vi "Dashboard Main.vi"() -> ()   [LabVIEW 2019]
uses:
  <vilib>/Utility/miscctls.llb/LVRowAndColumnTypeDef.ctl
  <vilib>/event_ctls.llb/eventvkey.ctl
  <vilib>/Rock Robotics/Network Tables/NT Read Numeric Array.vi
  <vilib>/Rock Robotics/WPI/Dashboard/WPI_DashboardLogging Global.vi
  <vilib>/Rock Robotics/Network Tables/NT Read Boolean.vi
panel:
  in  "Camera Settings Right":T1={"Frame Rate"=30, "Compression"=30, "Size"=1, "DB Camera Config"=FALSE} {"Frame Rate" scale=1.0..30.0; "Compression" scale=100.0..-1.0; "Size" items=["640x480", "320x240", "160x120"]}
  in  "Camera Name Right":string(combo)="No Camera Selection"
  out "Camera Perf":string
  in  "Camera Settings":T1={"Frame Rate"=30, "Compression"=30, "Size"=1, "DB Camera Config"=FALSE} {"Frame Rate" scale=1.0..30.0; "Compression" scale=100.0..-1.0; "Size" items=["640x480", "320x240", "160x120"]}
  in  "TCP":refnum<k5>
  in  "Rec Mode":enum32{"Stop", "Record", "Playback"}(radio)
  out "Robot IP":string
  out "Image Message":string="Timeout in Camera Communications"
  in  "Dashboard Tab":T2(tab)
  out "Vision Enabled":bool
  in  "Select Auto":string(combo)="Select Autonomous ..."
  out "NT Connection":bool
  out "MotorChart R":cluster{"Numeric":dbl, "Numeric":dbl}(graph)
  out "MotorChart L":cluster{"Numeric":dbl, "Numeric":dbl}(graph)
  out "MotorSliders R":cluster{"MotorSlide1":dbl, "MotorSlide2":dbl} {"MotorSlide2" scale=-1.0..1.0 scale format="%#_2e"; "MotorSlide1" scale=-1.0..1.0 scale format="%#_2e"}
  out "MotorSliders L":cluster{"MotorSlide1":dbl, "MotorSlide2":dbl} {"MotorSlide2" scale=-1.0..1.0 scale format="%#_2e"; "MotorSlide1" scale=-1.0..1.0 scale format="%#_2e"}
  out "JS1 Z":dbl(slide) scale=-1.0..1.0 scale format="%#_2e"
  out "JS1 Graph":cluster{"X":dbl, "Y":dbl}[](graph)
  out "JS1 Buttons":T3
  out "JS2 Z":dbl(slide) scale=-1.0..1.0 scale format="%#_2e"
  out "JS2 Graph":cluster{"X":dbl, "Y":dbl}[](graph)
  out "JS2 Buttons":T3
  out "Mode":T4(ring)=enum."Auto Disabled"
  out "Right Camera Perf":cluster{"Bandwidth (Mbps)":dbl, "FPS":dbl}
  out "Top RPM":dbl caption="DB/String 1"
  out "Bottom RPM":dbl caption="DB/String 1"
  out "Target Distance":dbl
  out "Camera Image Right":T5(plugin-control)
  out "Skew":dbl caption="DB/String 1"
  out "Area":dbl caption="DB/String 1"
  out "Offset X":dbl
  out "Offset Y":dbl
  in  "Test Slider":dbl(slide) scale=0.0..100.0 scale format="%#_3g"
  in  "On/Off":bool caption="Solenoid"
  in  "Test Name":u16(ring) items=["Select the test to run..."]
  in  "Test Tree":string(tree)
  in  "Motor":cluster{"Value":dbl, "Enable":bool} {"Value" scale=-1.0..1.0 scale format="%#_3g"}
  out "Progress":T6 {"Test Progress" scale=0.0..100.0}
  in  "Rev/Fwd":cluster{"Forward":bool, "Reverse":bool}
  in  "Test Ring":u16(ring) items=["Monochrome", "Color"]
  out "Cmd Status":string
  in  "Execute Command":bool
  in  "Command Params":string[][](table)
  in  "Command Selection":i32(listbox)
  in  "CheckList":i32(listbox)
  out "Tree":string(tree)
  out "Camera Image":T5(plugin-control)
  out "Background":bool
  in  "Camera Name":string(combo)="No Camera Selection"
  # "HW"
  # "HW"
  # "Drive Motors"
  # "Front"
  # "Operator 1"
  # "Operator 2"
  # "Right"
  # "Left"
  # "Back"
  # "This tab is a great place for autonomous settings and robot-specific values.\nPlace controls and indicators inside this tab and match name to\nDashboard Variables on robot. You can also delete this comment."
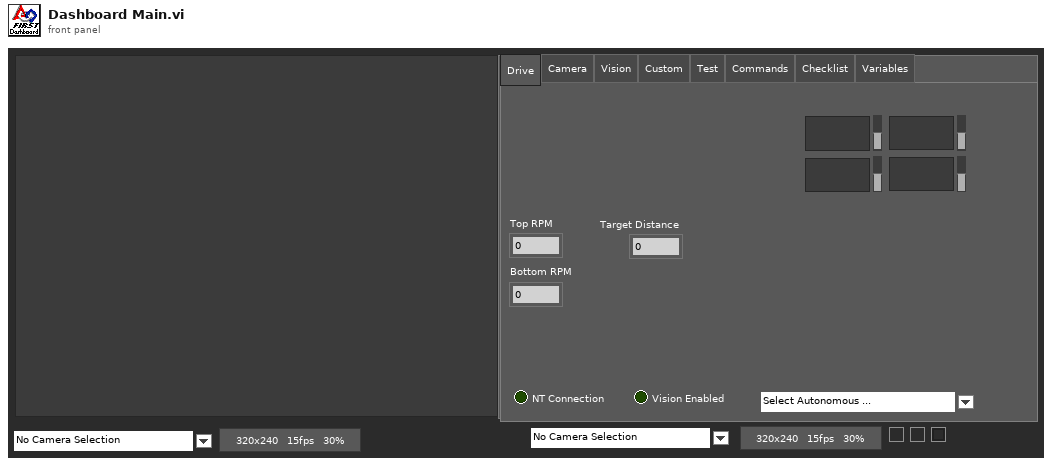
[diagram p1: front panel]
types:
  T1 = cluster{"Frame Rate":i32, "Compression":i32, "Size":u16, "DB Camera Config":bool}
  T2 = enum32{"Drive", "Camera", "Vision", "Custom", "Test", "Commands", "Checklist", "Variables"}
  T3 = cluster{bool, bool, bool, bool, bool, bool, bool, bool, bool, bool, bool, bool}
  T4 = enum8{"Tele-Op Disabled", "Tele-Op Enabled", "Auto Disabled", "Auto Enabled", "Test Disabled", "Test Enabled", "Disconnected", "No Code", "E-Stop"}
  T5 = typedef "IMAQ Image.ctl" = refnum<image>
  T6 = cluster{"Test Progress":u8, "Test Progress Text":string}
  T7 = cluster{"Save Path":path, "Interval (s)":dbl, "Keep":i32}
  T8 = enum32{"Drive", "Camera", "Basic", "Custom", "Test", "Commands", "Checklist", "Variables"}
  T9 = typedef "Image Type" = u32
  T10 = cluster{"IDs":cluster{"RPC field ID":u16, "Unique ID":u16}, "String":string}
  T11 = cluster{"Camera Image":refnum<vi>, "Dashboard Tab":refnum<vi>, "Background":refnum<vi>, "Rec Mode":refnum<vi>, "Test Slider":refnum<vi>, "On/Off ":refnum<vi>, "Test Ring":refnum<vi>, "Rev/Fwd":refnum<vi>, "Test Name":refnum<vi>, "Motor":refnum<vi>, "Progress":refnum<vi>, "CheckList":refnum<vi>, "Tree":refnum<vi>, "Test Tree":refnum<vi>, "Command Params":refnum<vi>, "Command Selection":refnum<vi>, "Execute Command":refnum<vi>, "Cmd Status":refnum<vi>, "Camera Settings":refnum<vi>, "Camera Name":refnum<vi>, "Camera Perf":refnum<vi>, "Camera Settings Right":refnum<vi>, "Camera Name Right":refnum<vi>, "Camera Image Right":refnum<vi>}
  T12 = cluster{"Global Rectangle":i32[], "Contours":cluster{"Contour Type":u32, "ROI Type":u32, "Points":i32[]}[]}
  T13 = cluster{"Camera Name Right":string, string, "Saved DB Images Info":cluster{"Save Path":path, "Interval (s)":dbl, "Keep":i32}}
  T14 = cluster{"Error Strings":string, "Disable Counts":cluster{u16, u16}, "Rail Faults":cluster{u16, u16, u16}, "Robot IP":string, "DB Mode":u8, "Event Info":cluster{"Name":string, "Type":u8, "Number":u16, "Replay":u8}}
  T15 = cluster{"Storage":cluster{"Disk Free":u64, "RAM Block":u32, "RAM free":u32}, "CPU Utilization":cluster{"CPU % ISR":sgl, "CPU % Time Crit":sgl, "CPU % Timed Str":sgl, "CPU % High":sgl, "CPU % Above":sgl, "CPU % Normal":sgl, "CPU % Low":sgl}, "CAN":cluster{"% Bus Utilization":sgl, "Bus Off Cnt":u32, "TX_FIFO Full Cnt":u32, "Receive Error Cnt":u8, "Transmit Error Cnt":u8}, "HID":cluster{"HID Outputs":u32, "Rumble Low":u16, "Rumble High":u16}[]}
  T16 = cluster{"Status bits":cluster{"Test Mode":bool, "Autonomous":bool, "Enabled":bool, "Code Start":bool, "Brownout":bool, "Reserved 2":bool, "Reserved 3":bool, "E-Stop":bool}, "Code Trace":cluster{"Disabled":bool, "TeleOp":bool, "Auto":bool, "Test":bool}, "Controller Type":enum16{"unknown", "cRIO", "roboRio"}, "Code?":enum16{"unknown", "noCode", "code"}, "Battery V":dbl}
  T17 = cluster{"Control Bits":cluster{"TestMode":bool, "Autonomous":bool, "Enabled":bool, "FMS Present":bool, bool, bool, bool, "E-Stop":bool}, "Team Station ":u8, "Countdown":sgl, "Joystick Values":cluster{"Axes":dbl[], "Buttons":bool[], "POVs":i16[]}[]}
  T18 = cluster{"Axes":dbl[], "Buttons":bool[], "POVs":i16[]}[]
  T19 = cluster{"Axes":dbl[], "Buttons":bool[], "POVs":i16[]}
  T20 = cluster{"Buttons[0]":bool, "Buttons[1]":bool, "Buttons[2]":bool, "Buttons[3]":bool, "Buttons[4]":bool, "Buttons[5]":bool, "Buttons[6]":bool, "Buttons[7]":bool, "Buttons[8]":bool, "Buttons[9]":bool, "Buttons[10]":bool, "Buttons[11]":bool}
  T21 = cluster{"Camera Name":string, string, "Saved DB Images Info":cluster{"Save Path":path, "Interval (s)":dbl, "Keep":i32}}
  T22 = cluster{"Operation":enum16{"Update", "Clear"}, "Color Box":u32}[]
  T23 = typedef "eventvkey.ctl" = enum16{"ASCII", "Enter", "Return", "Shift", "Ctrl", "Alt", "Cmd", "Opt", "Caps", "NumLock", "Clear", "Break", "Up", "Down", "Left", "Right", "Insert", "Delete", "Home", "End", "PageUp", "PageDown", "Escape", "Help", "Pause", "ScrollLock", "F1", "F2", "F3", "F4", "F5", "F6", "F7", "F8", "F9", "F10", "F11", "F12", "F13", "F14", "F15", "F16", "F17", "F18", "F19", "F20", "F21", "F22", "F23", "F24", "Play", "VolumeUp", "VolumeDown", "Mute", "Two Byte Char"}
  T24 = cluster{"Image Size":bool, "Image Type":bool, "Pixel Value":bool, "ROI Information":bool, "Zoom Factor":bool}
  T25 = cluster{"Operation":enum16{"Update", "Clear"}, "Color Box":u32}
  T26 = typedef "LVRowAndColumnTypeDef.ctl" = cluster{"Row":i32, "Column":i32}
  T27 = cluster{"Shift":bool, "Ctrl":bool, "Alt":bool, "Cmd":bool, "Opt":bool}
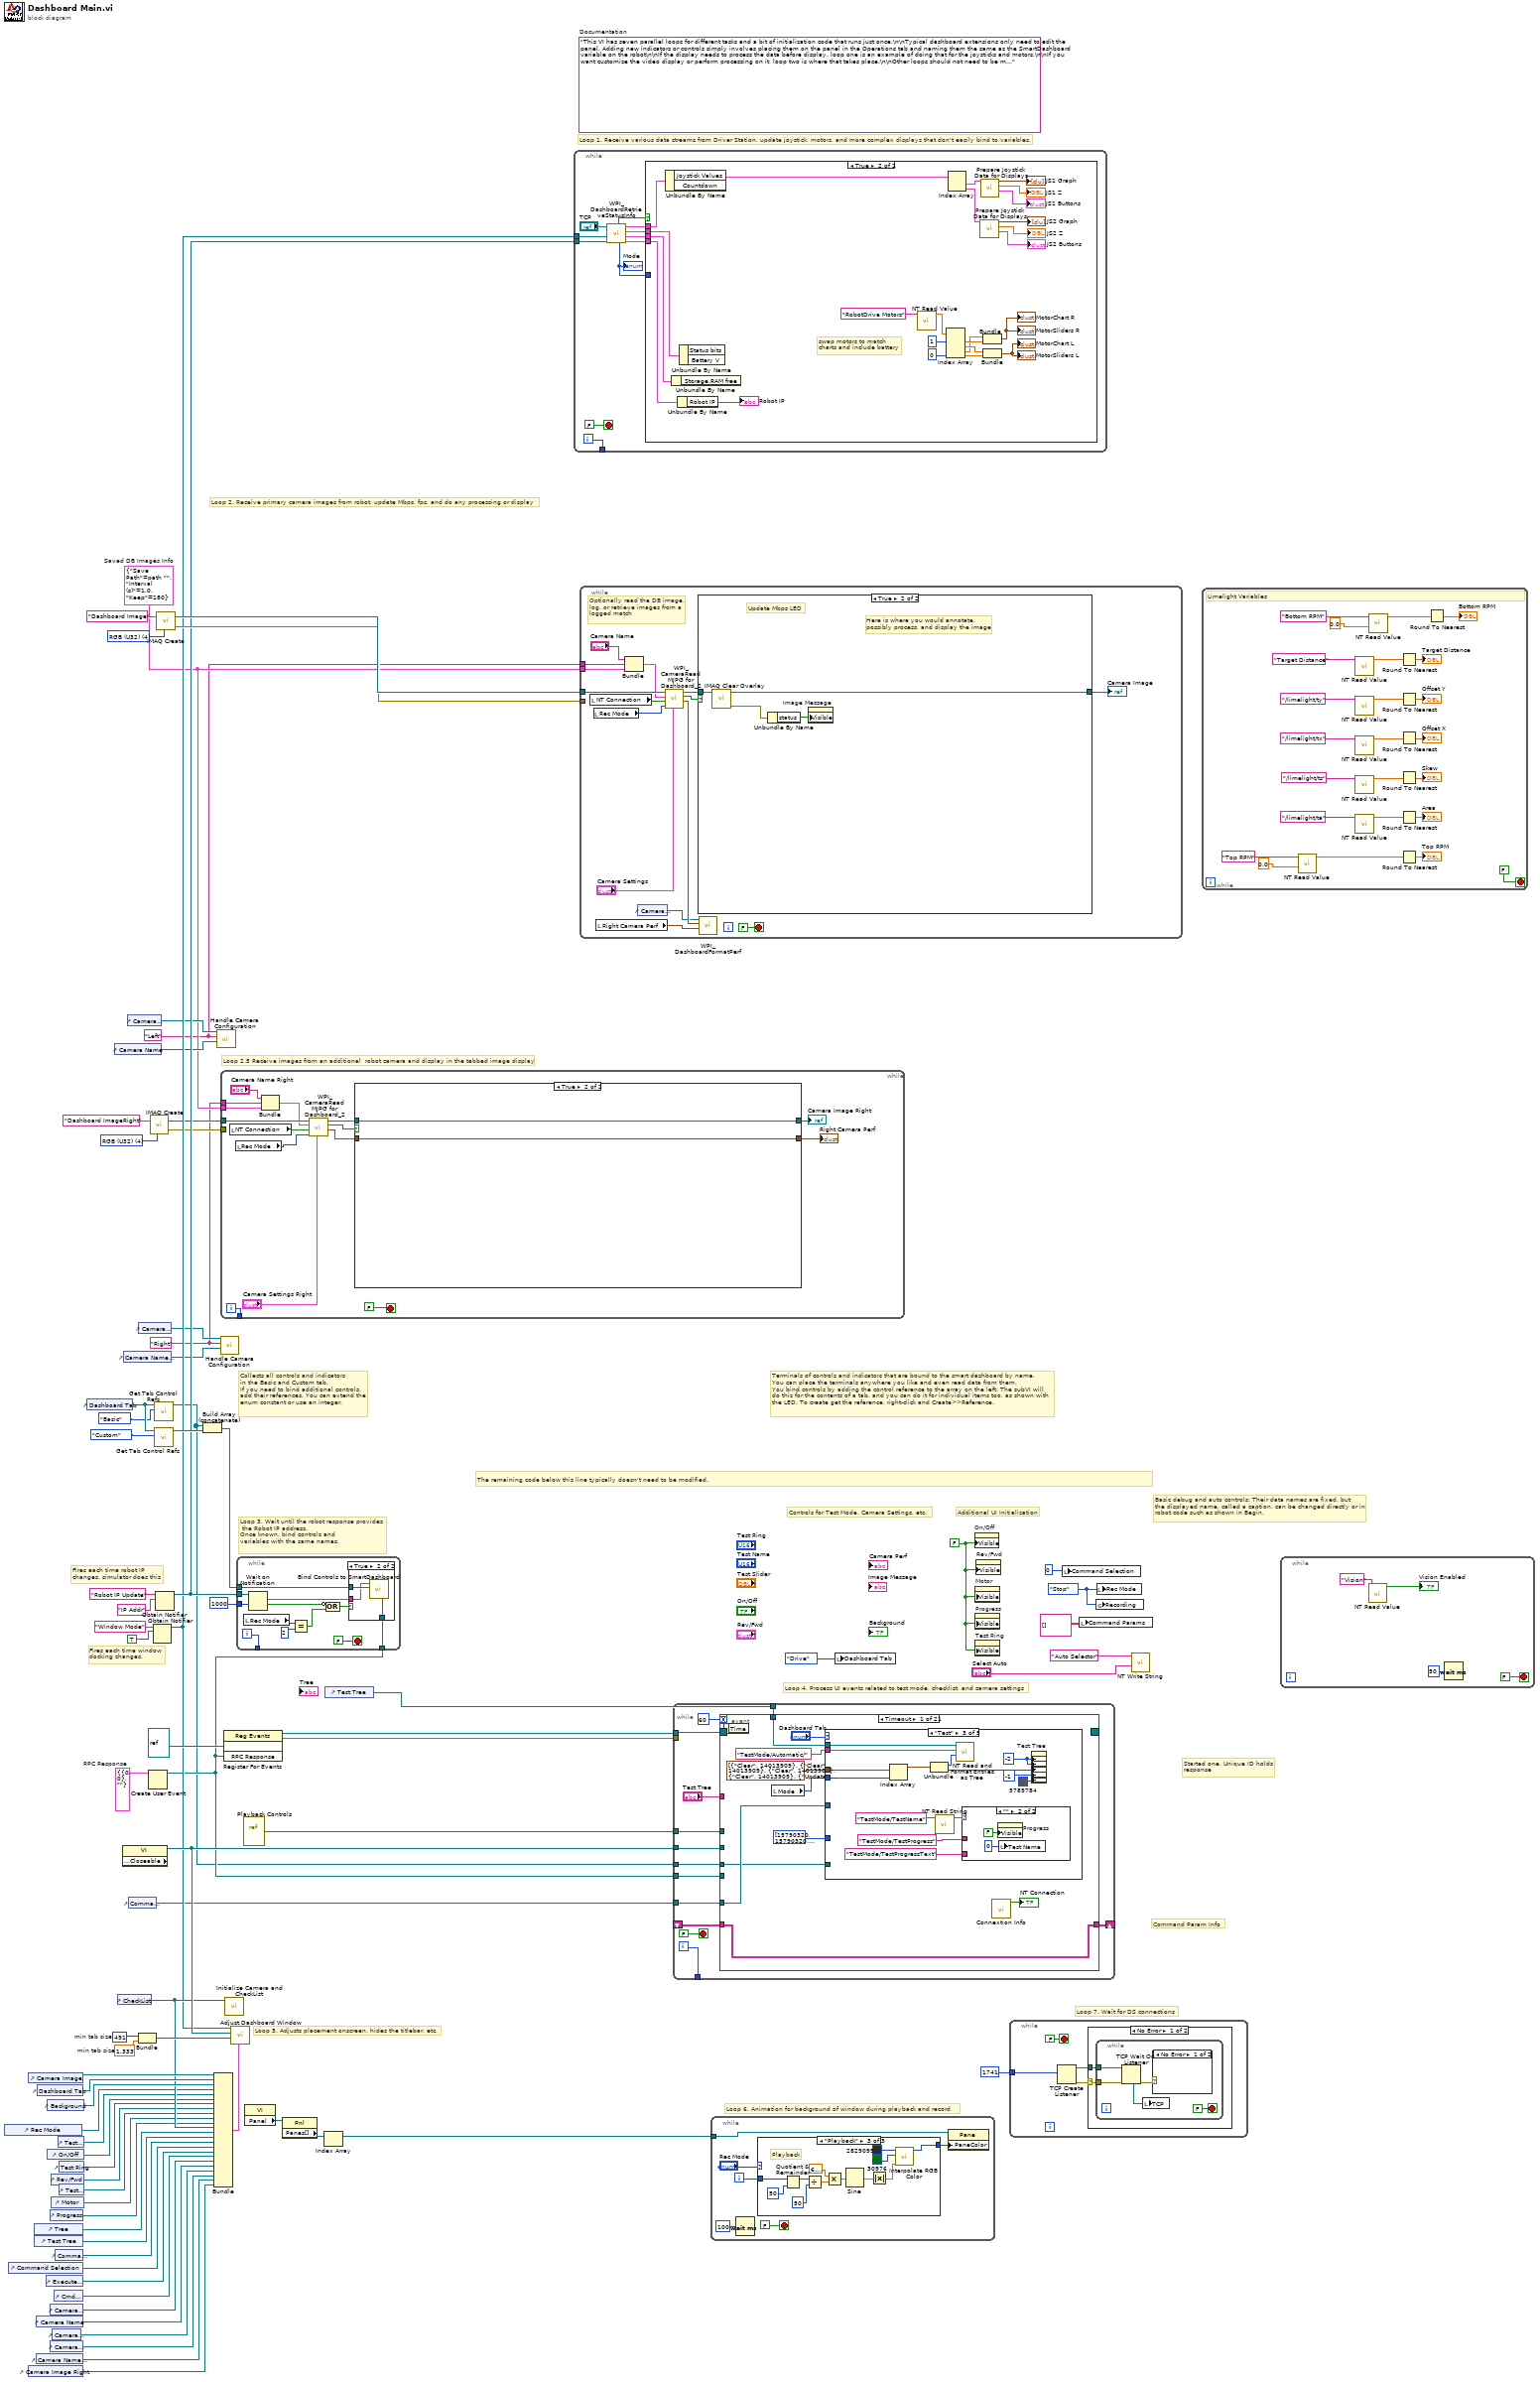
[diagram p0: block diagram]
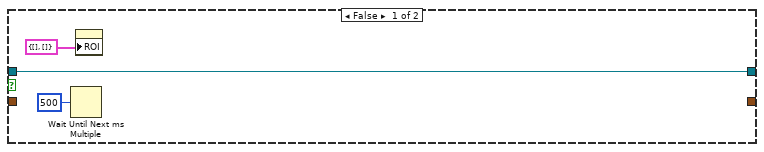
[diagram p2: hidden frame]
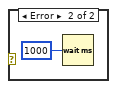
[diagram p3: hidden frame]
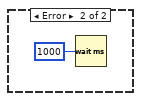
[diagram p4: hidden frame]
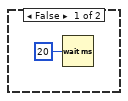
[diagram p5: hidden frame]
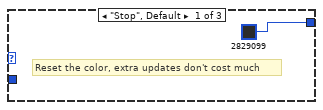
[diagram p6: hidden frame]
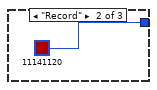
[diagram p7: hidden frame]
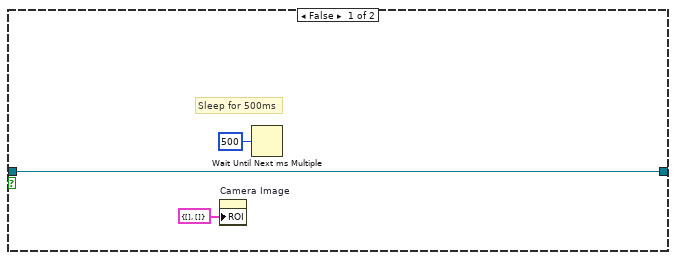
[diagram p9: hidden frame]
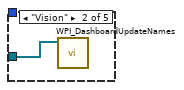
[diagram p11: hidden frame]
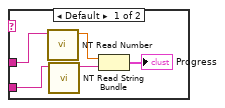
[diagram p12: hidden frame]
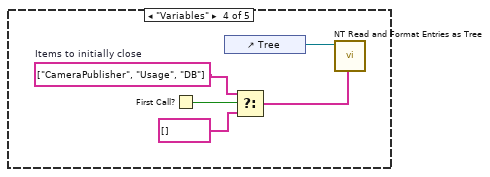
[diagram p13: hidden frame]
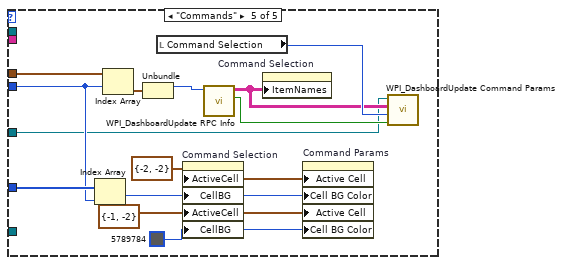
[diagram p14: hidden frame]
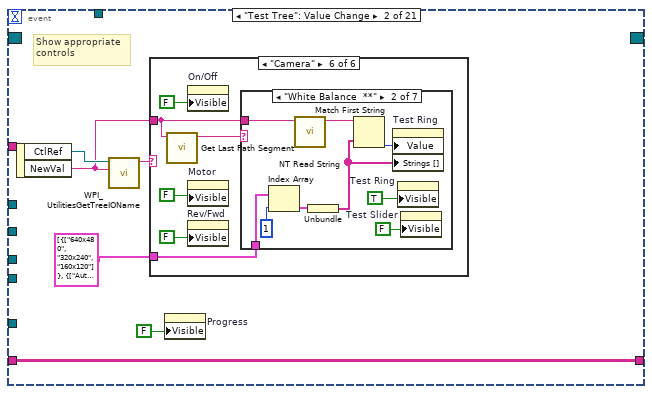
[diagram p15: hidden frame]
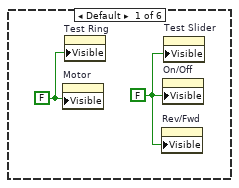
[diagram p16: hidden frame]
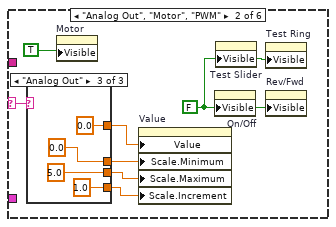
[diagram p17: hidden frame]
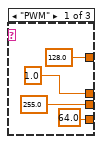
[diagram p18: hidden frame]
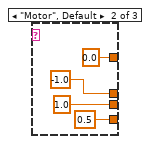
[diagram p19: hidden frame]
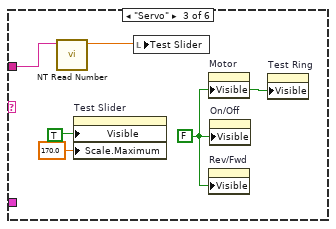
[diagram p20: hidden frame]
diagram:
  w4 = T7 {"Save Path"=path "", "Interval (s)"=1.0, "Keep"=180}  # Saved DB Images Info
  w3 = "Right"
  w2 = "Left"
  w14 = T9 4 items=["Grayscale (U8)", "Grayscale (I16)", "Grayscale (SGL)", "Complex (CSG)", "RGB (U32)", "HSL (U32)", "RGB (U64)"] ("Image Type")
  w30 = T10 {"IDs"={"RPC field ID"=0, "Unique ID"=0}, "String"=""}  # RPC Response
  w52 = 491  # min tab size
  w51 = 1.333  # min tab size
  w59 = enum32{"Stop", "Record", "Playback"}."Stop" ("Rec Mode")
  w36 = FALSE ("Visible")
  (unwired) "This VI has seven parallel loops for different tasks and a bit of initialization code that runs just once.\n\nTypical dashboard extensions only need to edit the panel. Adding new indicators or controls simply involves placing them on the panel in the Operations tab and naming them the same as the SmartDashboard variable on the robot\n\nIf the display needs to process the data before display, loop one is an example of doing that for the joysticks and motors.\n\nIf you want customize the video display or perform processing on it, loop two is where that takes place.\n\nOther loops should not need to be modified. They are pretty standard, and document the task they perform."  # Documentation
  w76 = T9 4 items=["Grayscale (U8)", "Grayscale (I16)", "Grayscale (SGL)", "Complex (CSG)", "RGB (U32)", "HSL (U32)", "RGB (U64)"] ("Image Type")
  # "Loop 2.5 Receive images from an additional  robot camera and display in the tabbed image display"
  # "Command Param Info"
  # "Started one, Unique ID holds\nresponse"
  # "Loop 7. Wait for DS connections"
  # "Basic debug and auto controls: Their data names are fixed, but\nthe displayed name, called a caption, can be changed directly or in\nrobot code such as shown in Begin."
  # "Controls for Test Mode, Camera Settings, etc."
  # "Additional UI Initialization"
  # "Loop 6. Animation for background of window during playback and record"
  # "Fires each time robot IP\nchanges, simulator does this"
  # "Fires each time window\ndocking changes."
  # "Collects all controls and indicators\nin the Basic and Custom tab.\nIf you need to bind additional controls,\nadd their references. You can extend the\nenum constant or use an integer."
  # "The remaining code below this line typically doesn't need to be modified."
  # "Loop 4. Process UI events related to test mode, checklist, and camera settings"
  # "Terminals of controls and indicators that are bound to the smart dashboard by name.\nYou can place the terminals anywhere you like and even read data from them.\nYou bind controls by adding the control reference to the array on the left. The subVI will\ndo this for the contents of a tab, and you can do it for individual items too, as shown with\nthe LED. To create get the reference, right-click and Create>>Reference."
  # "Loop 3. Wait until the robot response provides\n the Robot IP address.\nOnce known, bind controls and\nvariables with the same names."
  # "Loop 5. Adjusts placement onscreen, hides the titlebar, etc."
  # "Loop 1. Receive various data streams from Driver Station, update joystick, motors, and more complex displays that don't easily bind to variables."
  # "Loop 2. Receive primary camera images from robot, update Mbps, fps, and do any processing or display"
  n1 = control-ref of="Rec Mode"() -> (w42:refnum<vi>)
  n2 = control-ref of="Command Selection"() -> (w29:refnum<vi>)
  n3 = control-ref of="Camera Image Right"() -> (w7:refnum<vi>)
  n4 = control-ref of="Camera Image"() -> (w54:refnum<vi>)
  n5 = control-ref of="Tree"() -> (w46:refnum<vi>)
  n6 = control-ref of="Test Tree"() -> (w45:refnum<vi>)
  n7 = control-ref of="Camera Name"() -> (w20:refnum<vi>)
  n8 = control-ref of="Camera Name Right"() -> (w8:refnum<vi>)
  n9 = control-ref of="Dashboard Tab"() -> (w53:refnum<vi>)
  n10 = control-ref of="Execute Command"() -> (w31:refnum<vi>)
  n11 = control-ref of="Background"() -> (w49:refnum<vi>)
  n12 = control-ref of="On/Off"() -> (w40:refnum<vi>)
  n13 = control-ref of="Progress"() -> (w37:refnum<vi>)
  n14 = control-ref of="Camera Settings"() -> (w21:refnum<vi>)
  n15 = control-ref of="Camera Settings Right"() -> (w9:refnum<vi>)
  n16 = control-ref of="Rev/Fwd"() -> (w38:refnum<vi>)
  n17 = control-ref of="Motor"() -> (w43:refnum<vi>)
  n18 = control-ref of="Camera Perf"() -> (w19:refnum<vi>)
  n19 = control-ref of="Cmd Status"() -> (w25:refnum<vi>)
  n20 = control-ref of="Command Params"() -> (w32:refnum<vi>)
  n21 = control-ref of="Test Slider"() -> (w41:refnum<vi>)
  n22 = control-ref of="Test Ring"() -> (w39:refnum<vi>)
  n23 = control-ref of="Test Name"() -> (w44:refnum<vi>)
  n24 = control-ref of="Dashboard Tab"() -> (w57:refnum<vi>)
  n25 = control-ref of="Camera Name"() -> (w22:refnum<vi>)
  n26 = control-ref of="CheckList"() -> (w47:refnum<vi>)
  n27 = property class="VI" props=["Front Panel.Closeable"]() -> (reference out=w58:refnum<vi>)  [unwired: 2 in, 2 out]
  n28 = control-ref of="Camera Name Right"() -> (w10:refnum<vi>)
  n29 = control-ref of="Camera Settings"() -> (w23:refnum<vi>)
  n30 = control-ref of="Command Params"() -> (w24:refnum<vi>)
  n31 = control-ref of="Camera Settings Right"() -> (w11:refnum<vi>)
  n32 = Bundle("min tab size"=w52, "min tab size"=w51) -> (w50:cluster{"min tab size":i32, "min tab size":dbl})  [unwired: 1 in]
  n33 = Create User Event(user event datatype=w30) -> (user event=w26:refnum<user-event>)  [unwired: 1 in, 1 out]
  n34 = call "IMAQ Create"("Image Name"="Dashboard ImageRight", "Image Type"=w14) -> ("New Image"=w13:T5, "error out"=w12:errorcluster)  [unwired: 2 in, 1 out]
  n35 = Obtain Notifier(name (unnamed)="Window Mode", notification data type=TRUE) -> (notifier out=w34:refnum<notifier>)  [unwired: 2 in, 2 out]
  n36 = call <vilib>:"Get Tab Control Refs.vi"("Page Index"=T8."Basic" ("Dashboard Tab"), "TabControl in"=w57) -> ("ControlsOnPage"=w18:refnum<vi>[])  [unwired: 9 in]
  n37 = call <vilib>:"Get Tab Control Refs.vi"("Page Index"=T8."Custom" ("Dashboard Tab"), "TabControl in"=w57) -> ("ControlsOnPage"=w56:refnum<vi>[])  [unwired: 9 in]
  n38 = Obtain Notifier(name (unnamed)="Robot IP Update", notification data type="IP Addr" ("name (unnamed)")) -> (notifier out=w35:refnum<notifier>)  [unwired: 2 in, 2 out]
  n39 = call "IMAQ Create"("Image Name"="Dashboard Image", "Image Type"=w76) -> ("New Image"=w74:T5, "error out"=w73:errorcluster)  [unwired: 2 in, 1 out]
  n40 = Build Array (concatenate)(w18, w56) -> (w55:refnum<vi>[])
  n41 = Bundle("Camera Image"=w54, "Dashboard Tab"=w53, "Background"=w49, "Rec Mode"=w42, "Test Slider"=w41, "On/Off"=w40, "Test Ring"=w39, "Rev/Fwd"=w38, "Test Name"=w44, "Motor"=w43, "Progress"=w37, "CheckList"=w47, "Tree"=w46, "Test Tree"=w45, "Command Params"=w32, "Command Selection"=w29, "Execute Command"=w31, "Cmd Status"=w25, "Camera Settings"=w21, "Camera Name"=w20, "Camera Perf"=w19, "Camera Settings Right"=w9, "Camera Name Right"=w8, "Camera Image Right"=w7) -> (w48:T11)  [unwired: 1 in]
  n42 = call "Handle Camera Configuration.vi"("CameraNameRef"=w22, "Display Name"=w2, "ClusterRef"=w23) -> ()  [unwired: 9 in]
  n43 = call "Handle Camera Configuration.vi"("CameraNameRef"=w10, "Display Name"=w3, "ClusterRef"=w11) -> ()  [unwired: 9 in]
  n44 = while {
    tunnel: w13 -> [w91]
    tunnel: w12 -> [_]
    tunnel: [w86] -> _
    tunnel: w4 -> [w83]
    tunnel: w3 -> [w80]
    i -> [w86]
    stop <- FALSE stop-if-true
    n45 = local read "NT Connection"() -> (w84:bool)
    n46 = local read "Rec Mode"() -> (w90:enum32{"Stop", "Record", "Playback"})
    n47 = Bundle("Camera Name Right"="Camera Name Right", w80, "Saved DB Images Info"=w83) -> (w82:T13)  [unwired: 1 in]
    n48 = call <vilib>:"WPI_CameraRead MJPG for Dashboard_2.vi"("Camera Settings"="Camera Settings Right", "Rec Mode"=w90, "NT Connection"=w84, "Capture Info"=w82, "Image in"=w91) -> ("perf info"=w78:cluster{"Bandwidth (Mbps)":dbl, "fps":dbl}, "Active"=w85:bool, "Image\\ out"=w88:T5)  [unwired: 4 in]
    n49 = case shown="True" w85 {
      tunnel: w88 -> [w93 w95]
      tunnel: [w93 w95] -> w77
      tunnel: [_ w96] -> w79
      tunnel: w78 -> [_ w96]
      frame False {
        n50 = Wait Until Next ms Multiple(millisecond multiple=u32 500) -> ()  [unwired: 1 out]
        n51 = property on="Camera Image Right" class="ImageControl"("ROI"=T12 {"Global Rectangle"=[], "Contours"=[]}) -> ()  [unwired: 2 in, 2 out]
      }
      frame True {
      }
    }
    "Right Camera Perf" <- w79
    "Camera Image Right" <- w77
  }
  n52 = register-events(refnum<vi> refnum, w26) -> (reference out=w63:refnum<event-registration>, error out=w62:errorcluster)  [unwired: 2 in]
  n53 = call "Initialize Camera and CheckList.vi"("ListBox in"=w47) -> ()  [unwired: 11 in]
  n54 = call "Adjust Dashboard Window.vi"("Sizing Refnums"=w48, "Size Constraints"=w50, "VI"=w58, "WIn Mode"=w34) -> ()  [unwired: 8 in]
  n55 = while {
    tunnel: w55 -> [w108]
    tunnel: w35 -> [w106]
    tunnel: [w104] -> _
    tunnel: u32 1000 ("milliseconds to wait") -> [w103]
    tunnel: w26 -> [w97]
    i -> [w104]
    stop <- FALSE stop-if-true
    n56 = local read "Rec Mode"() -> (w99:enum32{"Stop", "Record", "Playback"})
    n57 = Wait on Notification(notifier=w106, timeout in ms (-1)=w103) -> (notification=w105:string, timed out?=w101:bool)  [unwired: 2 in, 2 out]
    n58 = Equal?(x=w99, y=u16 2 ("Rec Mode")) -> (x = y?=w100:bool)
    n59 = Compound Arithmetic op=OR(invert w101, w100) -> (w102:bool)
    n60 = case shown="True" w102 {
      tunnel: w108 -> [_ w111]
      tunnel: w105 -> [_ w110]
      tunnel: w97 -> [_ w109]
      frame False {
      }
      frame True {
        n61 = call <vilib>:"Bind Controls to SmartDashboard.vi"("RPC ref"=w109, "Bound Control Refs"=w111, "Server IP Address"=w110) -> ()  [unwired: 9 in]
      }
    }
  }
  n62 = vi-ref "Playback Controls.vi"() -> (w64:refnum<vi>)
  n63 = property class="VI"() -> ("Panel"=w66:refnum<vi>)  [unwired: 2 in, 2 out]
  n64 = property class="Pnl"(reference=w66) -> ("Panes[]"=w67:refnum<vi>[])  [unwired: 1 in, 2 out]
  n65 = Index Array(array=w67) -> (element=w65:refnum<vi>)  [unwired: 1 in]
  n66 = control-ref of="Test Tree"() -> (w68:refnum<vi>)
  n67 = while {
    tunnel: [w121] -> _
    tunnel: w35 -> [w115]
    tunnel: w34 -> [w112]
    i -> [w121]
    stop <- FALSE stop-if-true
    n68 = call <vilib>:"WPI_DashboardRetrieveStatusInfo.vi"("Binding Refnum"=w115, "Window Mode Notifier"=w112, "TCP Cnx"="TCP") -> ("Power and Errors"=w116:T14, "Robot Metrics"=w119:T15, "Status Info"=w120:T16, "Control Info"=w117:T17, "Robot Mode"=w114:T4, "Process?"=w118:bool)  [unwired: 3 in]
    "Mode" <- w114
    n69 = case shown="True" w118 {
      tunnel: w120 -> [_ w147]
      tunnel: w119 -> [_ w146]
      tunnel: w117 -> [_ w145]
      tunnel: w116 -> [_ w144]
      tunnel: w114 -> [_ _]
      frame False {
        n70 = Wait (ms)(milliseconds to wait=u32 20) -> ()  [unwired: 1 out]
      }
      frame True {
        # "swap motors to match\ncharts and include battery"
        n71 = Unbundle By Name(w145) -> ("Joystick Values"=w135:T18)  [unwired: 1 out]
        n72 = Unbundle By Name(w146) -> ()  [unwired: 1 out]
        n73 = Unbundle By Name(w144) -> ("Robot IP"=→"Robot IP":string)
        n74 = Unbundle By Name(w147) -> ()  [unwired: 2 out]
        n75 = call-poly <vilib>:"NT Read Value.vi"("Name"="RobotDrive Motors") -> ("Numeric Array"=w125:dbl[])  [unwired: 9 in, 1 out]
        n76 = Index Array(array=w125, index #1=1, index #4=0) -> (element #1=w139:dbl, element #2=w140:dbl, element #3=w138:dbl, element #4=w143:dbl)  [unwired: 2 in]
        n77 = Index Array(array=w135) -> (element #1=w134:T19, element #2=w130:T19)  [unwired: 2 in]
        n78 = call "Prepare Joystick Data for Displays.vi"("Joystick Values"=w130) -> ("Buttons"=→"JS2 Buttons":T20, "Z Axis"=→"JS2 Z":dbl, "Cartesian Data"=→"JS2 Graph":cluster{"X axis":dbl, "X axis":dbl}[])  [unwired: 8 in]
        n79 = call "Prepare Joystick Data for Displays.vi"("Joystick Values"=w134) -> ("Buttons"=→"JS1 Buttons":T20, "Z Axis"=→"JS1 Z":dbl, "Cartesian Data"=→"JS1 Graph":cluster{"X axis":dbl, "X axis":dbl}[])  [unwired: 8 in]
        n80 = Bundle("Numeric"=w138, "Numeric"=w139) -> (→"MotorChart R" →"MotorSliders R":cluster{"Numeric":dbl, "Numeric":dbl})  [unwired: 1 in]
        n81 = Bundle("Numeric"=w140, "Numeric"=w143) -> (→"MotorChart L" →"MotorSliders L":cluster{"Numeric":dbl, "Numeric":dbl})  [unwired: 1 in]
      }
    }
  }
  n82 = while {
    tunnel: w74 -> [w161]
    tunnel: w73 -> [_]
    tunnel: w4 -> [w155]
    tunnel: w2 -> [w152]
    stop <- FALSE stop-if-true
    # "Optionally read the DB image,\nlog, or retrieve images from a\nlogged match"
    n83 = local read "NT Connection"() -> (w156:bool)
    n84 = local read "Rec Mode"() -> (w158:enum32{"Stop", "Record", "Playback"})
    n85 = local read "Right Camera Perf"() -> (w150:cluster{"Bandwidth (Mbps)":dbl, "FPS":dbl})
    n86 = Bundle("Camera Name"="Camera Name", w152, "Saved DB Images Info"=w155) -> (w154:T21)  [unwired: 1 in]
    n87 = control-ref of="Camera Perf"() -> (w149:refnum<vi>)
    n88 = call <vilib>:"WPI_CameraRead MJPG for Dashboard_2.vi"("Camera Settings"="Camera Settings", "Rec Mode"=w158, "NT Connection"=w156, "Capture Info"=w154, "Image in"=w161) -> ("perf info"=w151:cluster{"Bandwidth (Mbps)":dbl, "fps":dbl}, "Active"=w159:bool, "Image\\ out"=w160:T5)  [unwired: 4 in]
    n89 = case shown="True" w159 {
      tunnel: w160 -> [w164 w167]
      tunnel: [w164 w166] -> w148
      frame False {
        # "Sleep for 500ms"
        n90 = property on="Camera Image" class="ImageControl"("ROI"=T12 {"Global Rectangle"=[], "Contours"=[]}) -> ()  [unwired: 2 in, 2 out]
        n91 = Wait Until Next ms Multiple(millisecond multiple=u32 500) -> ()  [unwired: 1 out]
      }
      frame True {
        # "Here is where you would annotate,\npossibly process, and display the image"
        # "Update Mbps LED"
        n92 = call "IMAQ Clear Overlay"("Image"=w167) -> ("error out"=w168:errorcluster, "Image Out"=w166:T5)  [unwired: 2 in, 7 out]
        n93 = Unbundle By Name(w168) -> ("status"=w169:bool)
        n94 = property on="Image Message" class="Str"("Visible"=w169) -> ()  [unwired: 2 in, 2 out]
      }
    }
    "Camera Image" <- w148
    n95 = call <vilib>:"WPI_DashboardFormatPerf.vi"("Right Camera Perf"=w150, "Performance"=w151, "String in"=w149) -> ()  [unwired: 9 in]
  }
  n96 = while {
    tunnel: [w179] -> _
    tunnel: w68 -> [w178]
    tunnel: w64 -> [w177]
    tunnel: w63 -> [w176]
    tunnel: w62 -> [_]
    tunnel: w58 -> [w175]
    tunnel: w26 -> [w174]
    tunnel: w24 -> [w173]
    shift-right: [w172] -> _
    shift-left: _ -> [w171]
    tunnel: w18 -> [w170]
    i -> [w179]
    stop <- FALSE stop-if-true
    n97 = event shown="[0] Timeout" {
      selector: w176 -> [_ _ _ _ _ _ _ _ _ _ _ _ _ _ _ _ _ _ _ _ _]
      dyn-events: [_ _ _ _ _ _ _ _ _ _ _ _ _ _ _ _ w439 _ _ _ _] -> _
      timeout: u32 60 ("milliseconds to wait") -> [_ _ _ _ _ _ _ _ _ _ _ _ _ _ _ _ _ _ _ _ _]
      tunnel: w178 -> [w191 _ _ _ _ _ _ _ _ _ _ _ _ _ _ _ _ _ _ _ _]
      tunnel: "Test Tree" -> [_ _ _ _ _ _ _ _ _ _ _ w406 w414 w416 w420 w428 _ _ _ _ _]
      tunnel: w177 -> [_ _ _ _ _ _ _ _ _ _ _ _ _ _ _ _ w441 _ w459 _ _]
      tunnel: w175 -> [_ _ _ _ _ _ _ _ _ _ _ _ _ _ _ _ w437 _ _ _ _]
      tunnel: w174 -> [_ _ _ _ _ _ _ _ _ _ _ _ _ _ _ _ w435 _ _ _ _]
      tunnel: w173 -> [w186 _ _ _ _ _ w357 _ _ _ _ _ _ _ _ _ _ _ _ _ _]
      tunnel: [w185 w234 w336 w341 w350 w354 w355 w364 w374 w381 w393 w405 w412 w415 w419 w427 w434 w454 w456 w460 w473] -> w172
      tunnel: w171 -> [w185 w234 w336 w341 w350 w354 w355 _ _ w381 w393 w405 w412 w415 w419 w427 w434 w454 w456 w460 w473]
      tunnel: w170 -> [w183 _ _ _ _ _ _ _ _ _ _ _ _ _ _ _ _ _ _ _ _]
      event Timeout {
        n98 = event-data() -> ()  [unwired: 1 in, 1 out]
        n99 = local read "Mode"() -> (w188:T4)
        n100 = case shown="\"Test\"" "Dashboard Tab" {
          tunnel: w191 -> [_ _ w207 _ _]
          tunnel: "TestMode/Automatic/" ("Name Pattern") -> [_ _ w206 _ _]
          tunnel: T22 [{"Operation"=enum."Clear", "Color Box"=14013909}, {"Operation"=enum."Clear", "Color Box"=14013909}, {"Operation"=enum."Clear", "Color Box"=14013909}, {"Operation"=enum."Clear", "Color Box"=14013909}, {"Operation"=enum."Update", "Color Box"=14013909}, {"Operation"=enum."Update", "Color Box"=16777215}, {"Operation"=enum."Clear", "Color Box"=14013909}, {"Operation"=enum."Clear", "Color Box"=14013909}, {"Operation"=enum."Clear", "Color Box"=14013909}] -> [_ _ w199 _ w227]
          tunnel: w188 -> [_ _ w198 _ w226]
          tunnel: u32[] [15790320, 15790320, 15790320, 15790320, 16777215, 16777215, 15790320, 15790320, 15790320] -> [_ _ _ _ w232]
          tunnel: w186 -> [_ _ _ _ w220]
          tunnel: w183 -> [_ w193 _ _ _]
          frame "Custom", Default {
          }
          frame "Vision" {
            n101 = call <vilib>:"WPI_DashboardUpdateNames.vi"("Controls on Tab"=w193) -> ()  [unwired: 11 in]
          }
          frame "Test" {
            w205 = -2 ("Active Item:Row Number")
            n102 = Index Array(array=w199, index=w198) -> (element=w200:T25)
            n103 = Unbundle(w200) -> ("Operation"=w201:enum16{"Update", "Clear"}, "Color Box"=w202:u32)
            n104 = call <vilib>:"NT Read String.vi"("Name"="TestMode/TestName") -> ("String"=w196:string)  [unwired: 9 in, 1 out]
            n105 = call <vilib>:"NT Read and Format Entries as Tree.vi"("Operation"=w201, "Name Pattern"=w206, "Tree Refnum"=w207) -> ()  [unwired: 7 in, 2 out]
            n106 = case shown="\"\"" w196 {
              tunnel: "TestMode/TestProgress" ("Name") -> [w209 _]
              tunnel: "TestMode/TestProgressText" ("Name") -> [w208 _]
              frame Default {
                n107 = call <vilib>:"NT Read Number.vi"("Name"=w209) -> ("Numeric"=w210:dbl)  [unwired: 9 in, 1 out]
                n108 = call <vilib>:"NT Read String.vi"("Name"=w208) -> ("String"=w211:string)  [unwired: 9 in, 1 out]
                n109 = Bundle("Numeric"=w210, "String"=w211) -> (→"Progress":cluster{"Numeric":dbl, "String":string})  [unwired: 1 in]
              }
              frame "" {
                n110 = property on="Progress" class="Clust (strict)"("Visible"=FALSE) -> ()  [unwired: 2 in, 2 out]
                n111 = local write "Test Name"(u16 0) -> ()
              }
            }
            n112 = property on="Test Tree" class="Tree (strict)"("Active Item Row Number"=w205, "ActiveColNum"=w205, "CellBG"=w202, "Active Item Row Number"=-1 ("Active Item:Row Number"), "CellBG"=u32 5789784 ("Color Box")) -> ()  [unwired: 2 in, 2 out]
          }
          frame "Variables" {
            w217 = string[] ["CameraPublisher", "Usage", "DB"]  # Items to initially close
            n113 = First Call?() -> (First Call?: T/F=w218:bool)
            n114 = control-ref of="Tree"() -> (w219:refnum<vi>)
            n115 = Select(t=w217, s=w218, f=string[] []) -> (s? t:f=w215:string[])
            n116 = call <vilib>:"NT Read and Format Entries as Tree.vi"("Tags to  Close"=w215, "Tree Refnum"=w219) -> ()  [unwired: 8 in, 2 out]
          }
          frame "Commands" {
            w228 = u32 5789784 ("Color Box")
            w229 = T26 {"Row"=-1, "Column"=-2} ("Active Cell:Active Cell")
            w231 = T26 {"Row"=-2, "Column"=-2} ("Active Cell:Active Cell")
            n117 = Index Array(array=w232, index=w226) -> (element=w230:u32)
            n118 = Index Array(array=w227, index=w226) -> (element=w225:T25)
            n119 = Unbundle(w225) -> ("Operation"=w224:enum16{"Update", "Clear"})  [unwired: 1 out]
            n120 = local read "Command Selection"() -> (w223:i32)
            n121 = property on="Command Selection" class="MCListbox (strict)"("ActiveCell"=w231, "CellBG"=w230, "ActiveCell"=w229, "CellBG"=w228) -> ()  [unwired: 2 in, 2 out]
            n122 = call <vilib>:"WPI_DashboardUpdate RPC Info.vi"("Operation"=w224) -> ("update"=w222:bool, "commands"=w221:string[][])  [unwired: 9 in]
            n123 = property on="Command Selection" class="MCListbox (strict)"("ItemNames"=w221) -> ()  [unwired: 2 in, 2 out]
            n124 = property on="Command Params" class="Tbl (strict)"("Active Cell"=w231, "Cell BG Color"=w230, "Active Cell"=w229, "Cell BG Color"=w228) -> ()  [unwired: 2 in, 2 out]
            n125 = call <vilib>:"WPI_DashboardUpdate Command Params.vi"("Update"=w222, "NewVal"=w223, "Commands"=w221, "Param Tbl"=w220) -> ()  [unwired: 7 in, 1 out]
          }
        }
        n126 = call <vilib>:"Connextion Info.vi"() -> ("Connected"=→"NT Connection":bool)  [unwired: 10 in, 1 out]
      }
      event "Test Tree": Value Change {
        # "Show appropriate\ncontrols"
        n127 = event-data() -> ("CtlRef"=w237:refnum<vi>, "NewVal"=w235:string)  [unwired: 1 in]
        n128 = call <vilib>:"WPI_UtilitiesGetTreeIOName.vi"("NewVal"=w235, "TreeControl in"=w237) -> ("I/O Name"=w238:string)  [unwired: 9 in]
        n129 = case shown="\"Camera\"" w238 {
          selector: w238 -> [_ w245 _ w267 w276 _]
          tunnel: w235 -> [_ _ w264 w266 _ w283]
          tunnel: cluster{string[]}[] [{["640x480", "320x240", "160x120"]}, {["Auto", "Fixed indoor", "Fixed outdoor 1", "Fixed outdoor 2", "Fixed fluorescent 1", "Fixed fluorescent 2", "Hold current"]}, {["Auto", "Flicker-free 50 Hz", "Flicker-free 60 Hz", "Hold current"]}, {["None", "Prioritize frame rate", "Prioritize image quality"]}, {["Monochrome", "Color"]}] -> [_ _ _ _ _ w282]
          frame Default {
            w240 = FALSE ("Visible")
            w239 = FALSE ("Visible")
            n130 = property on="Motor" class="Clust (strict)"("Visible"=w239) -> ()  [unwired: 2 in, 2 out]
            n131 = property on="Test Ring" class="Ring (strict)"("Visible"=w239) -> ()  [unwired: 2 in, 2 out]
            n132 = property on="Rev/Fwd" class="Clust (strict)"("Visible"=w240) -> ()  [unwired: 2 in, 2 out]
            n133 = property on="On/Off" class="Bool (strict)"("Visible"=w240) -> ()  [unwired: 2 in, 2 out]
            n134 = property on="Test Slider" class="Slide (strict)"("Visible"=w240) -> ()  [unwired: 2 in, 2 out]
          }
          frame "Analog Out", "Motor", "PWM" {
            w246 = FALSE ("Visible")
            n135 = case shown="\"Analog Out\"" w245 {
              tunnel: [1.0 ("Value") -1.0 ("Value") 0.0 ("Value")] -> w244
              tunnel: [255.0 ("Value") 1.0 ("Value") 5.0 ("Value")] -> w243
              tunnel: [128.0 ("Value") 0.0 ("Value") 0.0 ("Value")] -> w242
              tunnel: [64.0 ("Value") 0.5 ("Value") 1.0 ("Value")] -> w241
              frame "PWM" {
              }
              frame "Motor", Default {
              }
              frame "Analog Out" {
              }
            }
            n136 = property on="Motor" class="Clust (strict)"("Visible"=TRUE) -> ()  [unwired: 2 in, 2 out]
            n137 = property on="Value" class="Slide (strict)"("Value"=w242, "Scale.Minimum"=w244, "Scale.Maximum"=w243, "Scale.Increment"=w241) -> ()  [unwired: 2 in, 2 out]
            n138 = property on="On/Off" class="Bool (strict)"("Visible"=w246) -> ()  [unwired: 2 in, 2 out]
            n139 = property on="Test Slider" class="Slide (strict)"("Visible"=w246) -> ()  [unwired: 2 in, 2 out]
            n140 = property on="Test Ring" class="Ring (strict)"("Visible"=w246) -> ()  [unwired: 2 in, 2 out]
            n141 = property on="Rev/Fwd" class="Clust (strict)"("Visible"=w246) -> ()  [unwired: 2 in, 2 out]
          }
          frame "Servo" {
            w262 = FALSE ("Visible")
            n142 = call <vilib>:"NT Read Number.vi"("Name"=w264) -> ("Numeric"=w263:dbl)  [unwired: 9 in, 1 out]
            n143 = property on="Test Slider" class="Slide (strict)"("Visible"=TRUE, "Scale.Maximum"=170.0 ("Scale.Range:Maximum")) -> ()  [unwired: 2 in, 2 out]
            n144 = local write "Test Slider"(w263) -> ()
            n145 = property on="Motor" class="Clust (strict)"("Visible"=w262) -> ()  [unwired: 2 in, 2 out]
            n146 = property on="Rev/Fwd" class="Clust (strict)"("Visible"=w262) -> ()  [unwired: 2 in, 2 out]
            n147 = property on="On/Off" class="Bool (strict)"("Visible"=w262) -> ()  [unwired: 2 in, 2 out]
            n148 = property on="Test Ring" class="Ring (strict)"("Visible"=w262) -> ()  [unwired: 2 in, 2 out]
          }
          frame "Relay", "Solenoid" {
            w265 = FALSE ("Visible")
            n149 = property on="Motor" class="Clust (strict)"("Visible"=w265) -> ()  [unwired: 2 in, 2 out]
            n150 = property on="Test Slider" class="Slide (strict)"("Visible"=w265) -> ()  [unwired: 2 in, 2 out]
            n151 = Search and Replace String(input string=w266, search string="/Value  **", replace string="/Direction") -> (result string=w272:string)  [unwired: 5 in, 3 out]
            n152 = property on="Test Ring" class="Ring (strict)"("Visible"=w265) -> ()  [unwired: 2 in, 2 out]
            n153 = call <vilib>:"NT Read String.vi"("Name"=w272) -> ("String"=w270:string)  [unwired: 9 in, 1 out]
            n154 = Equal?(x="Both directions", y=w270) -> (x = y?=w268:bool)
            n155 = Not(x=w268) -> (.not. x?=w269:bool)
            n156 = property on="Rev/Fwd" class="Clust (strict)"("Visible"=w268) -> ()  [unwired: 2 in, 2 out]
            n157 = property on="On/Off" class="Bool (strict)"("Visible"=w269, "Caption.Text"=w267) -> ()  [unwired: 2 in, 2 out]
          }
          frame "Compressor", "Digital Out" {
            w275 = FALSE ("Visible")
            # "Get direction and finish"
            n158 = property on="Motor" class="Clust (strict)"("Visible"=w275) -> ()  [unwired: 2 in, 2 out]
            n159 = property on="Test Slider" class="Slide (strict)"("Visible"=w275) -> ()  [unwired: 2 in, 2 out]
            n160 = property on="Test Ring" class="Ring (strict)"("Visible"=w275) -> ()  [unwired: 2 in, 2 out]
            n161 = property on="On/Off" class="Bool (strict)"("Visible"=TRUE, "Caption.Text"=w276) -> ()  [unwired: 2 in, 2 out]
            n162 = property on="Rev/Fwd" class="Clust (strict)"("Visible"=FALSE) -> ()  [unwired: 2 in, 2 out]
          }
          frame "Camera" {
            n163 = call <vilib>:"Get Last Path Segment.vi"("String in"=w283) -> ("String out"=w284:string)  [unwired: 10 in]
            n164 = property on="On/Off" class="Bool (strict)"("Visible"=FALSE) -> ()  [unwired: 2 in, 2 out]
            n165 = property on="Motor" class="Clust (strict)"("Visible"=FALSE) -> ()  [unwired: 2 in, 2 out]
            n166 = property on="Rev/Fwd" class="Clust (strict)"("Visible"=FALSE) -> ()  [unwired: 2 in, 2 out]
            n167 = case shown="\"White Balance  **\"" w284 {
              tunnel: w283 -> [w290 w299 w308 w317 w326 _ w332]
              tunnel: w282 -> [w288 w296 w305 w314 w323 _ _]
              frame "Size  **" {
                n168 = Index Array(array=w288) -> (element=w287:cluster{string[]})  [unwired: 1 in]
                n169 = call <vilib>:"NT Read String.vi"("Name"=w290) -> ("String"=w289:string)  [unwired: 9 in, 1 out]
                n170 = Unbundle(w287) -> (w285:string[])
                n171 = Match First String(2:w285, 3:w289) -> (0:w286:i32)  [unwired: 1 out]
                n172 = property on="Test Ring" class="Ring (strict)"("Value"=w286, "Strings []"=w285) -> ()  [unwired: 2 in, 2 out]
                n173 = property on="Test Ring" class="Ring (strict)"("Visible"=TRUE) -> ()  [unwired: 2 in, 2 out]
                n174 = property on="Test Slider" class="Slide (strict)"("Visible"=FALSE) -> ()  [unwired: 2 in, 2 out]
              }
              frame "White Balance  **" {
                n175 = Index Array(array=w296, index=1) -> (element=w297:cluster{string[]})
                n176 = call <vilib>:"NT Read String.vi"("Name"=w299) -> ("String"=w298:string)  [unwired: 9 in, 1 out]
                n177 = Unbundle(w297) -> (w294:string[])
                n178 = Match First String(2:w294, 3:w298) -> (0:w293:i32)  [unwired: 1 out]
                n179 = property on="Test Ring" class="Ring (strict)"("Value"=w293, "Strings []"=w294) -> ()  [unwired: 2 in, 2 out]
                n180 = property on="Test Ring" class="Ring (strict)"("Visible"=TRUE) -> ()  [unwired: 2 in, 2 out]
                n181 = property on="Test Slider" class="Slide (strict)"("Visible"=FALSE) -> ()  [unwired: 2 in, 2 out]
              }
              frame "Exposure  **" {
                n182 = Index Array(array=w305, index=2) -> (element=w306:cluster{string[]})
                n183 = call <vilib>:"NT Read String.vi"("Name"=w308) -> ("String"=w307:string)  [unwired: 9 in, 1 out]
                n184 = Unbundle(w306) -> (w302:string[])
                n185 = Match First String(2:w302, 3:w307) -> (0:w303:i32)  [unwired: 1 out]
                n186 = property on="Test Ring" class="Ring (strict)"("Value"=w303, "Strings []"=w302) -> ()  [unwired: 2 in, 2 out]
                n187 = property on="Test Ring" class="Ring (strict)"("Visible"=TRUE) -> ()  [unwired: 2 in, 2 out]
                n188 = property on="Test Slider" class="Slide (strict)"("Visible"=FALSE) -> ()  [unwired: 2 in, 2 out]
              }
              frame "Exposure Priority  **" {
                n189 = Index Array(array=w314, index=3) -> (element=w315:cluster{string[]})
                n190 = call <vilib>:"NT Read String.vi"("Name"=w317) -> ("String"=w316:string)  [unwired: 9 in, 1 out]
                n191 = Unbundle(w315) -> (w311:string[])
                n192 = Match First String(2:w311, 3:w316) -> (0:w312:i32)  [unwired: 1 out]
                n193 = property on="Test Ring" class="Ring (strict)"("Value"=w312, "Strings []"=w311) -> ()  [unwired: 2 in, 2 out]
                n194 = property on="Test Ring" class="Ring (strict)"("Visible"=TRUE) -> ()  [unwired: 2 in, 2 out]
                n195 = property on="Test Slider" class="Slide (strict)"("Visible"=FALSE) -> ()  [unwired: 2 in, 2 out]
              }
              frame "Color Enable  **" {
                n196 = Index Array(array=w323, index=4) -> (element=w324:cluster{string[]})
                n197 = call <vilib>:"NT Read String.vi"("Name"=w326) -> ("String"=w325:string)  [unwired: 9 in, 1 out]
                n198 = Unbundle(w324) -> (w320:string[])
                n199 = Match First String(2:w320, 3:w325) -> (0:w321:i32)  [unwired: 1 out]
                n200 = property on="Test Ring" class="Ring (strict)"("Value"=w321, "Strings []"=w320) -> ()  [unwired: 2 in, 2 out]
                n201 = property on="Test Ring" class="Ring (strict)"("Visible"=TRUE) -> ()  [unwired: 2 in, 2 out]
                n202 = property on="Test Slider" class="Slide (strict)"("Visible"=FALSE) -> ()  [unwired: 2 in, 2 out]
              }
              frame Default {
                n203 = property on="Test Ring" class="Ring (strict)"("Visible"=FALSE) -> ()  [unwired: 2 in, 2 out]
                n204 = property on="Test Slider" class="Slide (strict)"("Visible"=FALSE) -> ()  [unwired: 2 in, 2 out]
              }
              frame "Brightness  **", "Color Level  **", "Compression  **", "FPS  **", "Sharpness  **" {
                n205 = call <vilib>:"NT Read Number.vi"("Name"=w332) -> ("Numeric"=w331:dbl)  [unwired: 9 in, 1 out]
                n206 = local write "Test Slider"(w331) -> ()
                n207 = property on="Test Slider" class="Slide (strict)"("Visible"=TRUE, "Scale.Maximum"=100.0 ("Scale.Range:Maximum")) -> ()  [unwired: 2 in, 2 out]
                n208 = property on="Test Ring" class="Ring (strict)"("Visible"=FALSE) -> ()  [unwired: 2 in, 2 out]
              }
            }
          }
        }
        n209 = property on="Progress" class="Clust (strict)"("Visible"=FALSE) -> ()  [unwired: 2 in, 2 out]
      }
      event "Test Name": Mouse Enter {
        # "Populate the ring with the list of tests"
        n210 = event-data() -> ()  [unwired: 1 in, 1 out]
        n211 = call <vilib>:"NT Read String Array.vi"("Name"="TestMode/TestList") -> ("String Array"=w340:string[])  [unwired: 9 in, 1 out]
        n212 = Build Array (concatenate)("Select the test to run...", w340) -> (w339:string[])
        n213 = property on="Test Name" class="Ring (strict)"("Strings []"=w339) -> ()  [unwired: 2 in, 2 out]
      }
      event "Test Name": Value Change {
        w342 = FALSE ("Visible")
        # "Tell the robot the test name to run"
        n214 = event-data() -> ("NewVal"=w346:u16)  [unwired: 1 in]
        n215 = property on="Test Name" class="Ring (strict)"() -> ("Strings []"=w347:string[])  [unwired: 2 in, 2 out]
        n216 = local write "Progress"(T6 {"Test Progress"=0, "Test Progress Text"=""} ("Progress")) -> ()
        n217 = Index Array(array=w347, index=w346) -> (element=w345:string)
        n218 = call <vilib>:"NT Write String.vi"("String"=w345, "Name"="TestMode/TestName") -> ()  [unwired: 9 in, 1 out]
        n219 = property on="Progress" class="Clust (strict)"("Visible"=TRUE) -> ()  [unwired: 2 in, 2 out]
        n220 = property on="Motor" class="Clust (strict)"("Visible"=w342) -> ()  [unwired: 2 in, 2 out]
        n221 = property on="Test Slider" class="Slide (strict)"("Visible"=w342) -> ()  [unwired: 2 in, 2 out]
        n222 = property on="On/Off" class="Bool (strict)"("Visible"=w342) -> ()  [unwired: 2 in, 2 out]
        n223 = property on="Rev/Fwd" class="Clust (strict)"("Visible"=w342) -> ()  [unwired: 2 in, 2 out]
        n224 = property on="Test Ring" class="Ring (strict)"("Visible"=w342) -> ()  [unwired: 2 in, 2 out]
      }
      event "Select Auto": Mouse Enter {
        # "Populate the combo box with the list of autonomous options"
        n225 = event-data() -> ()  [unwired: 1 in, 1 out]
        n226 = call <vilib>:"NT Read String Array.vi"("Name"="Auto List") -> ("String Array"=w349:string[])  [unwired: 9 in, 1 out]
        n227 = property on="Select Auto" class="CmbBox"("Strings[]"=w349) -> ()  [unwired: 2 in, 2 out]
      }
      event "Select Auto": Value Change {
        # "User modified the Auto Selection. Write to NT variable so robot knows."
        n228 = event-data() -> ("NewVal"=w352:string)  [unwired: 1 in]
        n229 = call <vilib>:"NT Write String.vi"("String"=w352, "Name"="Auto Selector") -> ()  [unwired: 9 in, 1 out]
      }
      event "Command Selection": Value Change {
        # "Get the params and show in table"
        n230 = event-data() -> ("NewVal"=w358:i32)  [unwired: 1 in]
        n231 = property on="Command Selection" class="MCListbox (strict)"() -> ("ItemNames"=w356:string[][])  [unwired: 2 in, 2 out]
        n232 = call <vilib>:"WPI_DashboardUpdate Command Params.vi"("NewVal"=w358, "Commands"=w356, "Param Tbl"=w357) -> ()  [unwired: 8 in, 1 out]
      }
      event "Execute Command": Value Change {
        # "Started one, Unique ID holds\nresponse"
        n233 = event-data() -> ()  [unwired: 1 in, 1 out]
        n234 = property on="Command Selection" class="MCListbox (strict)"() -> ("ItemNames"=w369:string[][])  [unwired: 2 in, 2 out]
        n235 = Index Array(array=w369, index (row)="Command Selection", index (col)=0) -> (element=w367:string)
        n236 = call <vilib>:"Invoke Commands.vi"("Command Params"="Command Params", "Function Name"=w367) -> ("Params"=w363:u8, "Started"=w362:bool)  [unwired: 7 in, 1 out]
        n237 = Array Subset(array="Command Params", length (row)=w363) -> (w364:string[][])  [unwired: 3 in]
        n238 = Select(t="Executing" ("Cmd Status"), s=w362, f="" ("Cmd Status")) -> (s? t:f=→"Cmd Status":string)
      }
      event "Command Selection": Double Click {
        n239 = event-data() -> ("Row"=w377:i32)  [unwired: 1 in]
        n240 = property on="Command Selection" class="MCListbox (strict)"() -> ("ItemNames"=w380:string[][])  [unwired: 2 in, 2 out]
        n241 = local read "Command Params"() -> (w376:string[][])
        n242 = Index Array(array=w380, index (row)=w377, index (col)=0) -> (element=w378:string)
        n243 = call <vilib>:"Invoke Commands.vi"("Command Params"=w376, "Function Name"=w378) -> ("Params"=w375:u8, "Started"=w370:bool)  [unwired: 7 in, 1 out]
        n244 = Array Subset(array=w376, length (row)=w375) -> (w374:string[][])  [unwired: 3 in]
        n245 = Select(t="Executing" ("Cmd Status"), s=w370, f="" ("Cmd Status")) -> (s? t:f=w371:string)
        n246 = local write "Cmd Status"(w371) -> ()
      }
      event "CheckList": Double Click {
        # "Shift clears all"
        # "Update symbols on the listbox"
        n247 = event-data() -> ("PlatMods.Shift"=w382:bool, "Row"=w384:i32)  [unwired: 1 in]
        n248 = case shown="True" w382 {
          tunnel: w384 -> [w388 _]
          tunnel: 1 -> [w387 _]
          frame False {
            n249 = property on="CheckList" class="LstBox (strict)"() -> ("Item Symbols"=w386:i32[])  [unwired: 2 in, 2 out]
            n250 = Replace Array Subset(array=w386, new element=w387, index=w388) -> (w385:i32[])
            n251 = property on="CheckList" class="LstBox (strict)"("Item Symbols"=w385) -> ()  [unwired: 2 in, 2 out]
          }
          frame True {
            w389 = 0 ("Top Row")
            n252 = property on="CheckList" class="LstBox (strict)"() -> ("Number of Rows"=w391:u32)  [unwired: 2 in, 2 out]
            n253 = Initialize Array(0, w391) -> (w390:i32[])
            n254 = property on="CheckList" class="LstBox (strict)"("Top Row"=w389, "Value"=w389, "Item Symbols"=w390) -> ()  [unwired: 2 in, 2 out]
          }
        }
      }
      event "CheckList": Key Down {
        # "Update symbols on the listbox\nLeft and right keys check and uncheck"
        n255 = event-data() -> ("VKey"=w395:T23)  [unwired: 1 in]
        n256 = case shown="\"Left\", \"Right\"" w395 {
          selector: w395 -> [w400 _]
          tunnel: eventvkey."Left" ("VKey") -> [w398 _]
          frame "Left", "Right" {
            n257 = Equal?(x=w398, y=w400) -> (x = y?=w399:bool)
            n258 = Select(t=0, s=w399, f=1) -> (s? t:f=w401:i32)
            n259 = property on="CheckList" class="LstBox (strict)"() -> ("Item Symbols"=w404:i32[])  [unwired: 2 in, 2 out]
            n260 = Replace Array Subset(array=w404, new element=w401, index="CheckList") -> (w403:i32[])
            n261 = property on="CheckList" class="LstBox (strict)"("Item Symbols"=w403) -> ()  [unwired: 2 in, 2 out]
          }
          frame Default {
          }
        }
      }
      event "Motor.Enable": Value Change {
        # "When the test mode otor enable helper is set, update that\ntree row item's value"
        n262 = event-data() -> ("NewVal"=w410:bool)  [unwired: 1 in]
        n263 = Unbundle("Motor") -> ("Value"=w409:dbl)  [unwired: 1 out]
        n264 = Select(t=w409, s=w410, f=0.0) -> (s? t:f=w407:dbl)
        n265 = call <vilib>:"NT Write Number.vi"("Numeric"=w407, "Name"=w406) -> ()  [unwired: 9 in, 1 out]
      }
      event "Test Slider": Value Change {
        # "When the test mode slider helper is set, update that\ntree row item's value"
        n266 = event-data() -> ("NewVal"=w413:dbl)  [unwired: 1 in]
        n267 = call <vilib>:"NT Write Number.vi"("Numeric"=w413, "Name"=w414) -> ()  [unwired: 9 in, 1 out]
      }
      event "On/Off": Value Change {
        # "When the test mode on/off helper value is set, update that\ntree row item's value"
        n268 = event-data() -> ("NewVal"=w418:bool)  [unwired: 1 in]
        n269 = Boolean To (0,1)(Boolean=w418) -> (0, 1=w417:i16)
        n270 = call <vilib>:"NT Write Number.vi"("Numeric"=w417, "Name"=w416) -> ()  [unwired: 9 in, 1 out]
      }
      event "Rev/Fwd": Value Change {
        # "When the test mode helper value for relays is set, update that\ntree row item's value"
        n271 = event-data() -> ("NewVal.Forward"=w426:bool, "NewVal.Reverse"=w425:bool)  [unwired: 1 in]
        n272 = Boolean To (0,1)(Boolean=w426) -> (0, 1=w422:i16)
        n273 = Boolean To (0,1)(Boolean=w425) -> (0, 1=w424:i16)
        n274 = Negate(x=w424) -> (-x=w423:i16)
        n275 = Add(x=w422, y=w423) -> (x+y=w421:i16)
        n276 = call <vilib>:"NT Write Number.vi"("Numeric"=w421, "Name"=w420) -> ()  [unwired: 9 in, 1 out]
      }
      event "Test Ring": Value Change {
        # "When a test mode helper value is selected from the ring,\nset the tree item's variable to the string value"
        n277 = event-data() -> ("NewVal"=w430:u16)  [unwired: 1 in]
        n278 = property on="Test Ring" class="Ring (strict)"() -> ("Strings []"=w431:string[])  [unwired: 2 in, 2 out]
        n279 = Index Array(array=w431, index=w430) -> (element=w429:string)
        n280 = call <vilib>:"NT Write String.vi"("String"=w429, "Name"=w428) -> ()  [unwired: 9 in, 1 out]
      }
      event "Rec Mode": Value Change {
        # "Update globals for recording mode and path to read log from.\nClear when logging and let NetworkTables set path for vision to\nuse."
        n281 = event-data() -> ("NewVal"=w442:enum32{"Stop", "Record", "Playback"})  [unwired: 1 in]
        n282 = global write "WPI_DashboardLogging Global.vi" "Logging Filename"(path "") -> ()
        n283 = global write "WPI_DashboardLogging Global.vi" "Recording"(w442) -> ()
        n284 = case shown="\"Playback\"" w442 {
          tunnel: w441 -> [_ w444 w453]
          tunnel: [_ _ w452] -> w439
          tunnel: [_ _ w451] -> _
          tunnel: w437 -> [_ _ w449]
          tunnel: cluster{i32, i32} {-250, 170} -> [_ _ w448]
          tunnel: [_ _ T24 {"Image Size"=TRUE, "Image Type"=TRUE, "Pixel Value"=TRUE, "ROI Information"=TRUE, "Zoom Factor"=FALSE} ("Image Information Shown:All Elements")] -> w432
          tunnel: [_ _ TRUE ("Zoom Factor")] -> w433
          tunnel: w435 -> [_ _ w445]
          frame Default {
          }
          frame "Stop", "Record" {
            # "Place Window too"
            n285 = invoke class="VI" method="FP.Close"(reference=w444) -> (reference out=w443:refnum<vi>)  [unwired: 2 in, 2 out]
            n286 = invoke class="VI" method="Abort VI"(reference=w443) -> ()  [unwired: 2 in, 3 out]
          }
          frame "Playback" {
            n287 = call "Open Playback Panel.vi"("Offset"=w448, "DB VI Ref"=w449, "Playback in"=w453) -> ("Playback out"=w450:refnum<vi>)  [unwired: 8 in]
            n288 = register-events(w450, w445) -> (reference out=w452:refnum<event-registration>, error out=w451:errorcluster)  [unwired: 2 in]
          }
        }
        n289 = property on="Camera Image Right" class="ImageControl"("Image Information Shown"=w432, "Image Information Visible"=w433) -> ()  [unwired: 2 in, 2 out]
        n290 = property on="Camera Image" class="ImageControl"("Image Information Shown"=w432, "Image Information Visible"=w433) -> ()  [unwired: 2 in, 2 out]
        n291 = call <vilib>:"WPI_DashboardNT Log FieldName Cache.vi"("Operation"=enum16{"Lookup/Add", "Index", "Clear"}."Clear") -> ()  [unwired: 8 in, 3 out]
      }
      event Panel Close {
        w455 = enum32{"Stop", "Record", "Playback"}."Stop" ("Rec Mode")
        # "Playback window has been closed, abort"
        n292 = event-data() -> ()  [unwired: 1 in, 4 out]
        n293 = local write "Rec Mode"(w455) -> ()
        n294 = global write "WPI_DashboardLogging Global.vi" "Recording"(w455) -> ()
      }
      event Panel Close {
        # "Abort playback window and ourself"
        n295 = event-data() -> ()  [unwired: 1 in, 4 out]
        n296 = invoke class="VI" method="FP.Close"(reference=w459) -> (reference out=w458:refnum<vi>)  [unwired: 2 in, 2 out]
        n297 = invoke class="VI" method="Abort VI"(reference=w458) -> (error out=w457:errorcluster)  [unwired: 2 in, 2 out]
        n298 = invoke class="VI" method="Abort VI"(error in=w457) -> ()  [unwired: 2 in, 3 out]
      }
      event User Event {
        n299 = event-data() -> ("IDs"=w466:cluster{"RPC field ID":u16, "Unique ID":u16}, "String"=w465:string)  [unwired: 1 in]
        n300 = Bundle("IDs"=w466, "String"=w465) -> (w464:T10)  [unwired: 1 in]
        n301 = call <vilib>:"Retrieve RPC Response.vi"("RPC Response"=w464) -> ("Output"=w462:string[][])  [unwired: 10 in]
        n302 = Build Array (concatenate)(w460, w462) -> (w461:string[][])
        n303 = local write "Command Params"(w461) -> ()
        n304 = local write "Cmd Status"("" ("Cmd Status")) -> ()
      }
      event "Tree": Double Click {
        n305 = event-data() -> ("PlatMods"=w472:T27, "Tag"=w469:string)  [unwired: 1 in]
        n306 = Unbundle(w472) -> ("Shift"=w471:bool)  [unwired: 4 out]
        n307 = String Subset(string=w469, length (rest)=1 ("length (rest)")) -> (substring=w468:string)  [unwired: 1 in]
        n308 = Not(x=w471) -> (.not. x?=w470:bool)
        n309 = case shown="\"/\"" w468 {
          tunnel: w469 -> [_ w475]
          tunnel: w470 -> [_ w474]
          frame Default {
          }
          frame "/" {
            n310 = call <vilib>:"NT Update Persistence.vi"("Persistence"=w474, "Name"=w475) -> ()  [unwired: 9 in, 1 out]
          }
        }
      }
    }
  }
  n311 = while {
    tunnel: w65 -> [w477]
    i -> [w480]
    stop <- FALSE stop-if-true
    n312 = Wait (ms)(milliseconds to wait=u32 100) -> ()  [unwired: 1 out]
    n313 = case shown="\"Playback\"" "Rec Mode" {
      tunnel: w480 -> [_ _ w495]
      tunnel: [u32 2829099 ("Base Color") u32 11141120 ("Target Color") w484] -> w476
      frame "Stop", Default {
        # "Reset the color, extra updates don't cost much"
      }
      frame "Record" {
      }
      frame "Playback" {
        # "Playback"
        n314 = Quotient & Remainder(x=w495, y=u32 50 ("milliseconds to wait")) -> (x-y*floor(x/y)=w491:u32)  [unwired: 1 out]
        n315 = Divide(x=w491, y=u32 50 ("milliseconds to wait")) -> (x/y=w488:dbl)
        n316 = Multiply(x=6.283185307179586, y=w488) -> (x*y=w493:dbl)
        n317 = Sine(x=w493) -> (sin(x)=w492:dbl)
        n318 = Absolute Value(x=w492) -> (abs(x)=w485:dbl)
        n319 = call "Interpolate RGB Color.vi"("Proportion"=w485, "Target Color"=u32 30976, "Base Color"=u32 2829099) -> ("Result Color"=w484:u32)  [unwired: 8 in]
      }
    }
    n320 = property class="Pane"(reference=w477, "PaneColor"=w476) -> ()  [unwired: 1 in, 2 out]
  }
  n321 = local write "Dashboard Tab"(T2."Drive" ("Dashboard Tab")) -> ()
  n322 = property on="On/Off" class="Bool (strict)"("Visible"=w36) -> ()  [unwired: 2 in, 2 out]
  n323 = property on="Motor" class="Clust (strict)"("Visible"=w36) -> ()  [unwired: 2 in, 2 out]
  n324 = property on="Progress" class="Clust (strict)"("Visible"=w36) -> ()  [unwired: 2 in, 2 out]
  n325 = property on="Test Ring" class="Ring (strict)"("Visible"=w36) -> ()  [unwired: 2 in, 2 out]
  n326 = property on="Rev/Fwd" class="Clust (strict)"("Visible"=w36) -> ()  [unwired: 2 in, 2 out]
  n327 = while {
    tunnel: u16 1741 ("timeout ms (25000)") -> [w497]
    stop <- FALSE stop-if-true
    n328 = TCP Create Listener(10:w497) -> (0:w496:errorcluster, 3:w498:refnum<k5>)  [unwired: 4 in, 1 out]
    n329 = case shown="No Error" w496 {
      selector: w496 -> [w500 _]
      tunnel: w498 -> [w501 _]
      frame No Error {
        n330 = while {
          tunnel: w501 -> [w504]
          tunnel: w500 -> [w503]
          stop <- FALSE stop-if-true
          n331 = TCP Wait On Listener(8:w503, 11:w504) -> (0:w505:errorcluster, 4:w506:refnum<k5>)  [unwired: 2 in, 3 out]
          n332 = local write "TCP"(w506) -> ()
          n333 = case shown="No Error" w505 {
            frame No Error {
            }
            frame Error {
              n334 = Wait (ms)(milliseconds to wait=u32 1000) -> ()  [unwired: 1 out]
            }
          }
        }
      }
      frame Error {
        n335 = Wait (ms)(milliseconds to wait=u32 1000) -> ()  [unwired: 1 out]
      }
    }
  }
  n336 = local write "Command Selection"(u16 0 ("milliseconds to wait")) -> ()
  n337 = local write "Command Params"(string[][] [] ("Command Params")) -> ()
  n338 = global write "WPI_DashboardLogging Global.vi" "Recording"(w59) -> ()
  n339 = local write "Rec Mode"(w59) -> ()
  n340 = call <vilib>:"NT Write String.vi"("String"="Select Auto", "Name"="Auto Selector") -> ()  [unwired: 9 in, 1 out]
  n341 = while {
    stop <- FALSE stop-if-true
    # "Limelight Variables"
    n342 = call-poly <vilib>:"NT Read Value.vi"("Default Value"=0.0, "Name"="Top RPM") -> ("Numeric"=w524:dbl)  [unwired: 8 in, 1 out]
    n343 = call-poly <vilib>:"NT Read Value.vi"("Name"="Target Distance") -> ("Numeric"=w522:dbl)  [unwired: 9 in, 1 out]
    n344 = call-poly <vilib>:"NT Read Value.vi"("Name"="/limelight/ty") -> ("Numeric"=w518:dbl)  [unwired: 9 in, 1 out]
    n345 = call-poly <vilib>:"NT Read Value.vi"("Name"="/limelight/tx") -> ("Numeric"=w520:dbl)  [unwired: 9 in, 1 out]
    n346 = call-poly <vilib>:"NT Read Value.vi"("Name"="/limelight/ts") -> ("Numeric"=w516:dbl)  [unwired: 9 in, 1 out]
    n347 = call-poly <vilib>:"NT Read Value.vi"("Name"="/limelight/ta") -> ("Numeric"=w514:dbl)  [unwired: 9 in, 1 out]
    n348 = call-poly <vilib>:"NT Read Value.vi"("Default Value"=0.0, "Name"="Bottom RPM") -> ("Numeric"=w512:dbl)  [unwired: 8 in, 1 out]
    n349 = Round To Nearest(number=w522) -> (nearest integer value=→"Target Distance":dbl)
    n350 = Round To Nearest(number=w518) -> (nearest integer value=→"Offset Y":dbl)
    n351 = Round To Nearest(number=w520) -> (nearest integer value=→"Offset X":dbl)
    n352 = Round To Nearest(number=w516) -> (nearest integer value=→"Skew":dbl)
    n353 = Round To Nearest(number=w514) -> (nearest integer value=→"Area":dbl)
    n354 = Round To Nearest(number=w524) -> (nearest integer value=→"Top RPM":dbl)
    n355 = Round To Nearest(number=w512) -> (nearest integer value=→"Bottom RPM":dbl)
  }
  n356 = while {
    stop <- FALSE stop-if-true
    n357 = call-poly <vilib>:"NT Read Value.vi"("Name"="Vision") -> ("Boolean"=→"Vision Enabled":bool)  [unwired: 9 in, 1 out]
    n358 = Wait (ms)(milliseconds to wait=u32 50) -> ()  [unwired: 1 out]
  }
